vi "Zero Phase Filter (Cascade, DBL).vi"(10 "IIR Filter Cluster":T1 {"Forward Coefficients" format="%.4f"; "Reverse Coefficients" format="%.4f"}, 11 "X":dbl[](array[numeric])) -> (0 "error":i32, 3 "Filtered X":dbl[](array[numeric]))   [LabVIEW 2017, in "NI_AALBase.lvlib"]
doc: "Applies a zero phase filter to an input sequence <B>X</B>. Wire data to the <B>X</B> input to determine the polymorphic instance to use or manually select the instance."
uses:
  NI_AALBase.lvlib
  <resource>/lvanlys.dll
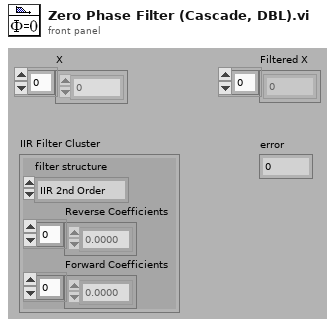
[diagram p1: front panel]
types:
  T1 = cluster{"filter structure":enum32{"IIR 2nd Order", "IIR 4th Order"}, "Reverse Coefficients":dbl[], "Forward Coefficients":dbl[]}
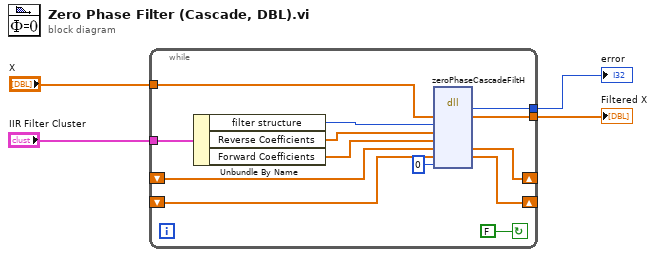
[diagram p0: block diagram]
diagram:
  n1 = while {
    tunnel: "X" -> [w17]
    tunnel: [w16] -> w3
    tunnel: "IIR Filter Cluster" -> [w12]
    tunnel: [w11] -> w1
    shift-right: [w10] -> _
    shift-left: _ -> [w9]
    shift-right: [w8] -> _
    shift-left: _ -> [w7]
    stop <- FALSE continue-if-true
    n2 = Unbundle By Name(w12) -> ("filter structure"=w15:enum32{"IIR 2nd Order", "IIR 4th Order"}, "Reverse Coefficients"=w14:dbl[], "Forward Coefficients"=w13:dbl[])
    n3 = dll-call lib="C:/Program Files (x86)/National Instruments/LabVIEW 2017/resource/lvanlys.*" fn="zeroPhaseCascadeFiltH"("xH"=w17, "stage_type"=w15, "aH"=w14, "bH"=w13, "s1H"=w9, "s2H"=w7, "reset"=0 ("init")) -> ("return type"=w11:i32, "xH"=w16:dbl[], "s1H"=w10:dbl[], "s2H"=w8:dbl[])  [unwired: 7 in, 2 out]
  }
  "Filtered X" <- w3
  "error" <- w1
